vi "CRYPEAQ RFFT.vi"(9 "ifn":i32=1, 10 "N":i32, 11 "x":dbl[](array[numeric])) -> (3 "X":dbl[](array[numeric]))   [LabVIEW 2013]
uses:
  <vilib>/Analysis/2dsp.llb/Inverse Real FFT.vi
  <vilib>/Analysis/2dsp.llb/Real FFT.vi
  <vilib>/Analysis/NI_AALPro.lvlib
panel:
  out "Numeric 2":dbl
  out "Numeric":dbl
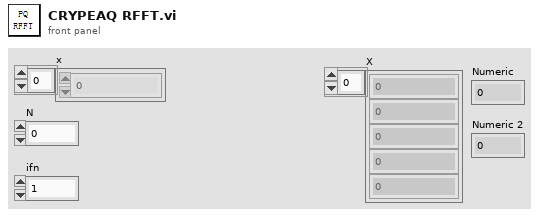
[diagram p1: front panel]
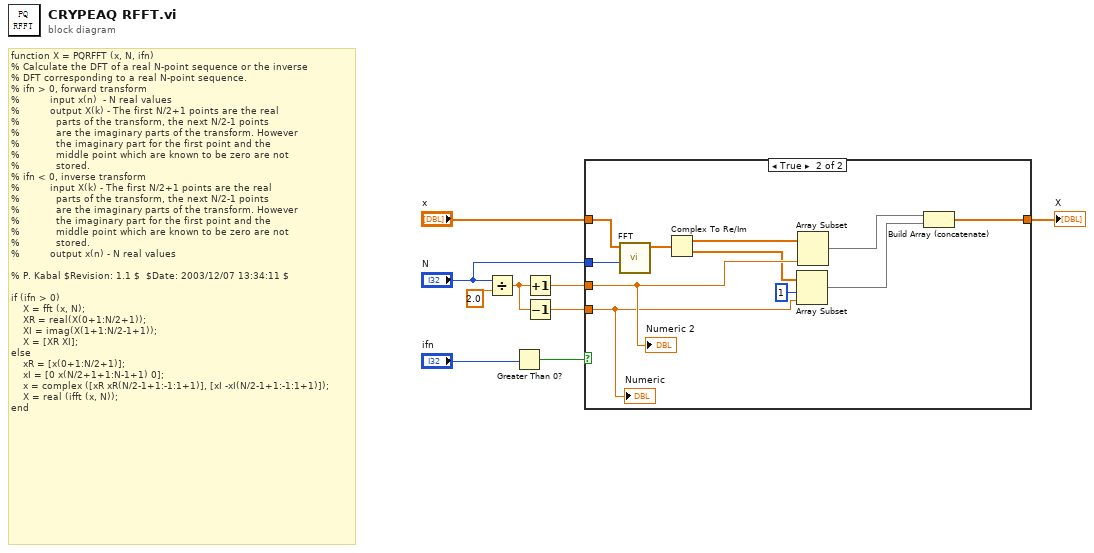
[diagram p0: block diagram]
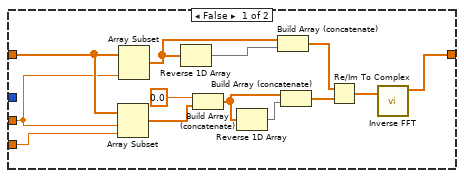
[diagram p2: hidden frame]
diagram:
  # "function X = PQRFFT (x, N, ifn)\n% Calculate the DFT of a real N-point sequence or the inverse\n% DFT corresponding to a real N-point sequence.\n% ifn > 0, forward transform\n%          input x(n)  - N real values\n%          output X(k) - The first N/2+1 points are the real\n%            parts of the transform, the next N/2-1 points\n%            are the imaginary parts of the transform. However\n%            the imaginary part for the first point and the\n%            middle point which are known to be zero are not\n%            stored.\n% ifn < 0, inverse transform\n%          input X(k) - The first N/2+1 points are the real\n%            parts of the transform, the next N/2-1 points\n%            are the imaginary parts of the transform. However\n%            the imaginary part for the first point and the\n%            middle point which are known to be zero are not\n%            stored.\n%          output x(n) - N real values\n\n% P. Kabal $Revision: 1.1 $  $Date: 2003/12/07 13:34:11 $\n\nif (ifn > 0)\n    X = fft (x, N);\n    XR = real(X(0+1:N/2+1));\n    XI = imag(X(1+1:N/2-1+1));\n    X = [XR XI];\nelse\n    xR = [x(0+1:N/2+1)];\n    xI = [0 x(N/2+1+1:N-1+1) 0];\n    x = complex ([xR xR(N/2-1+1:-1:1+1)], [xI -xI(N/2-1+1:-1:1+1)]);\n    X = real (ifft (x, N));\nend"
  n1 = Divide(x="N", y=2.0) -> (x/y=w6:dbl)
  n2 = Greater Than 0?(x="ifn") -> (x > 0?=w8:bool)
  n3 = Increment(x=w6) -> (x+1=w4:dbl)
  n4 = Decrement(x=w6) -> (x-1=w5:dbl)
  n5 = case shown="True" w8 {
    tunnel: "x" -> [w22 w33]
    tunnel: [w18 w32] -> w1
    tunnel: w4 -> [w17 w30]
    tunnel: w5 -> [w16 w27]
    tunnel: "N" -> [_ w29]
    frame False {
      n6 = Array Subset(array=w22, index=w17, length=w16) -> (w20:dbl[])
      n7 = Array Subset(array=w22, length=w17) -> (w15:dbl[])  [unwired: 1 in]
      n8 = Reverse 1D Array(array=w15) -> (reversed array=w14:dbl[])
      n9 = Build Array (concatenate)(0.0 ("element"), w20) -> (w12:dbl[])
      n10 = Reverse 1D Array(array=w12) -> (reversed array=w11:dbl[])
      n11 = Build Array (concatenate)(w15, w14) -> (w13:dbl[])
      n12 = Build Array (concatenate)(w12, w11) -> (w10:dbl[])
      n13 = Re/Im To Complex(1:w10, 2:w13) -> (0:w19:cdb[])
      n14 = call-poly <vilib>:"Inverse FFT.vi"("FFT {X}"=w19) -> ("X"=w18:dbl[])  [unwired: 9 in, 1 out]
    }
    frame True {
      n15 = call-poly <vilib>:"FFT.vi"("FFT size"=w29, "X"=w33) -> ("FFT {X}"=w28:cdb[])  [unwired: 1 in, 8 out]
      n16 = Complex To Re/Im(x + iy=w28) -> (x=w25:dbl[], y=w26:dbl[])
      n17 = Array Subset(array=w26, index=1, length=w27) -> (w23:dbl[])
      n18 = Array Subset(array=w25, length=w30) -> (w24:dbl[])  [unwired: 1 in]
      n19 = Build Array (concatenate)(w24, w23) -> (w32:dbl[])
      "Numeric" <- w27
      "Numeric 2" <- w30
    }
  }
  "X" <- w1
